vi "ccc_Convert To Compatibility TagConfig.vi"(11 "new tag":T1) -> (3 "old tag":T4)   [LabVIEW 2010]
uses:
  ccc_TagConfiguration.ctl
  <vilib>/NI/Current Value Table/Compatibility/_SubVIs/TypeDefs/cvt_Data Types.ctl
  ccc_TagDirection.ctl
  Tag Configuration.ctl
  <vilib>/NI/Current Value Table/Type Defs/Data Types.ctl
  Tag Direction.ctl
  <vilib>/NI/Current Value Table/Current Value Table.lvlib
  NI_CCC.lvlib
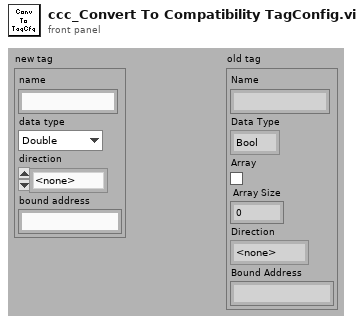
[diagram p1: front panel]
types:
  T1 = typedef "NI_CCC.lvlib/Tag Configuration.ctl" = cluster{"name":string, "data type":T2, "direction":T3, "bound address":string}
  T2 = typedef "Current Value Table.lvlib/Data Types.ctl" = enum16{"Double", "Single", "I64", "I32", "I16", "I8", "U64", "U32", "U16", "U8", "String", "Boolean"}
  T3 = typedef "NI_CCC.lvlib/Tag Direction.ctl" = enum32{"<none>", "Read", "Write"}
  T4 = typedef "ccc_TagConfiguration.ctl" = cluster{"Name":string, "Data Type":T5, "Array":bool, "Array Size":u32, "Direction":T6, "Bound Address":string}
  T5 = typedef "cvt_Data Types.ctl" = enum16{"Bool", "U8", "I32", "Double", "String", "Enum"}
  T6 = typedef "ccc_TagDirection.ctl" = enum32{"<none>", "Read", "Write"}
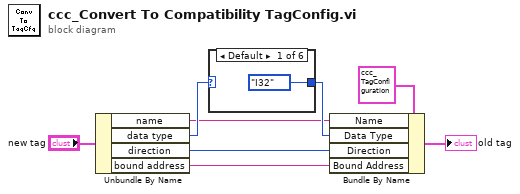
[diagram p0: block diagram]
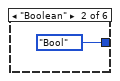
[diagram p2: hidden frame]
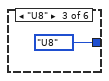
[diagram p3: hidden frame]
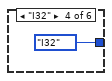
[diagram p4: hidden frame]
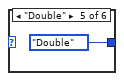
[diagram p5: hidden frame]
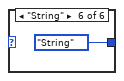
[diagram p6: hidden frame]
diagram:
  n1 = Unbundle By Name("new tag") -> ("name"=w3:string, "data type"=w6:T2, "direction"=w4:T3, "bound address"=w5:string)
  n2 = case shown="Default" w6 {
    tunnel: [cvt_Data_Types."I32" ("Data Type") cvt_Data_Types."Bool" ("Data Type") cvt_Data_Types."U8" ("Data Type") cvt_Data_Types."I32" ("Data Type") cvt_Data_Types."Double" ("Data Type") cvt_Data_Types."String" ("Data Type")] -> w8
    frame Default {
    }
    frame "Boolean" {
    }
    frame "U8" {
    }
    frame "I32" {
    }
    frame "Double" {
    }
    frame "String" {
    }
  }
  n3 = Bundle By Name(cluster=T4 {"Name"="", "Data Type"=enum."Bool", "Array"=FALSE, "Array Size"=0, "Direction"=enum."<none>", "Bound Address"=""} ("HMI DataEngine Tag List"), "Name"=w3, "Data Type"=w8, "Direction"=w4, "Bound Address"=w5) -> (→"old tag":T4)
